vi "ke37xx Reset Scan.vi"(0 "VISA Resource Name":refnum<visa-resource-name>, 11 "error in (no error)":errorcluster) -> (4 "VISA Resource Name Out":refnum<visa-resource-name>, 15 "error out":errorcluster)   [LabVIEW 2009, in "Keithley 3700 Series.lvlib"]
doc: "This VI resets the scanning aspects of the system to factory defaults."
uses:
  <instrlib>/Keithley 3706/Keithley 3700 Series.lvlib
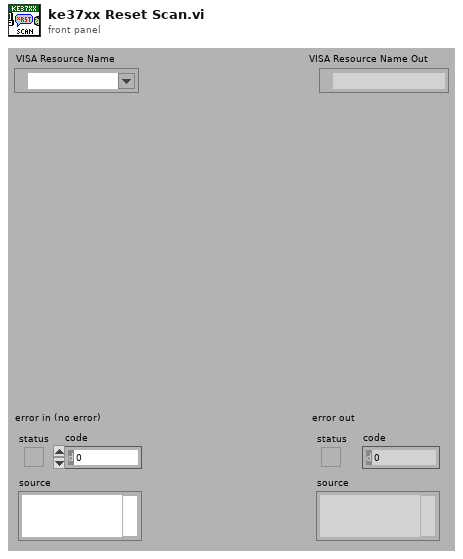
[diagram p1: front panel]
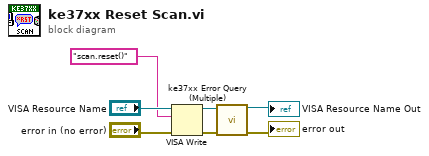
[diagram p0: block diagram]
diagram:
  n1 = VISA Write(VISA resource name="VISA Resource Name", write buffer="scan.reset()", error in (no error)="error in (no error)") -> (VISA resource name out=w3:refnum<visa-resource-name>, error out=w2:errorcluster)  [unwired: 1 out]
  n2 = call <instrlib>:"ke37xx Error Query (Multiple).vi"("VISA resource name"=w3, "error in (no error)"=w2) -> ("VISA resource name out"=→"VISA Resource Name Out":refnum<visa-resource-name>, "error out"=→"error out":errorcluster)  [unwired: 12 out]
